vi "ActorRefContainer Write Core.vi"(8 "error in (no error)":errorcluster, 10 "Core":T1, 11 "ActorRefContainer in":refnum<class "ActorRefContainer.lvclass">) -> (0 "error out":errorcluster, 3 "ActorRefContainer out":refnum<class "ActorRefContainer.lvclass">)   [LabVIEW 2019, in "ActorRefContainer.lvlib" / "ActorRefContainer.lvclass"]
uses:
  ActorRefContainer.lvclass
  <vilib>/ActorFramework/Message Enqueuer/Message Enqueuer.lvclass
  ActorRefContainer.lvclass/ActorRefContainer.ctl
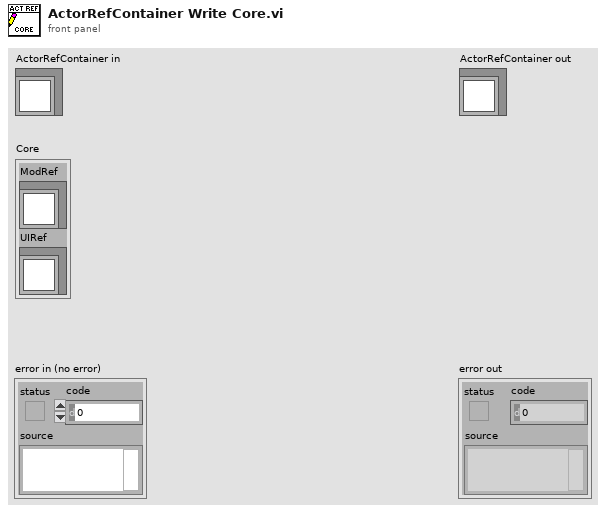
[diagram p1: front panel]
types:
  T1 = cluster{"ModRef":refnum<class "Message Enqueuer.lvclass">, "UIRef":refnum<class "Message Enqueuer.lvclass">}
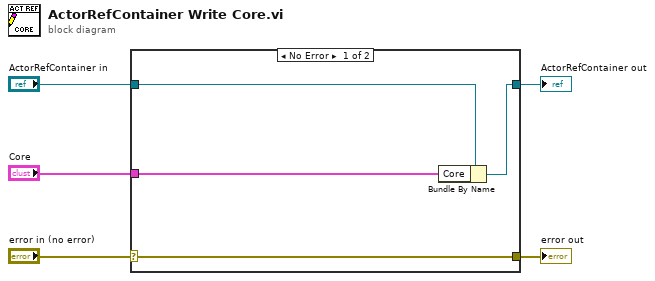
[diagram p0: block diagram]
diagram:
  n1 = case shown="No Error" "error in (no error)" {
    selector: "error in (no error)" -> [w9 w10]
    tunnel: [w9 w10] -> w4
    tunnel: [w7 w11] -> w2
    tunnel: "ActorRefContainer in" -> [w8 w11]
    tunnel: "Core" -> [w6 _]
    frame No Error {
      n2 = Bundle By Name(cluster=w8, "Core"=w6) -> (w7:refnum<class "ActorRefContainer.lvclass">)
    }
    frame Error {
    }
  }
  "error out" <- w4
  "ActorRefContainer out" <- w2
